vi "populate_database.vi"(11 "output cluster":T1) -> ()   [LabVIEW 2014]
uses:
  Program Files (x86)/National Instruments/LabVIEW 2014/vi.lib/addons/database/Connection.llb/DB Tools Open Connec (String).vi
  Program Files (x86)/National Instruments/LabVIEW 2014/vi.lib/addons/database/Connection.llb/Conn Execute.vi
  Program Files (x86)/National Instruments/LabVIEW 2014/vi.lib/addons/database/Recordset.llb/Rec Destroy - Connection.vi
  Program Files (x86)/National Instruments/LabVIEW 2014/vi.lib/addons/database/NI_Database_API.lvlib
panel:
  out "resulting string":string
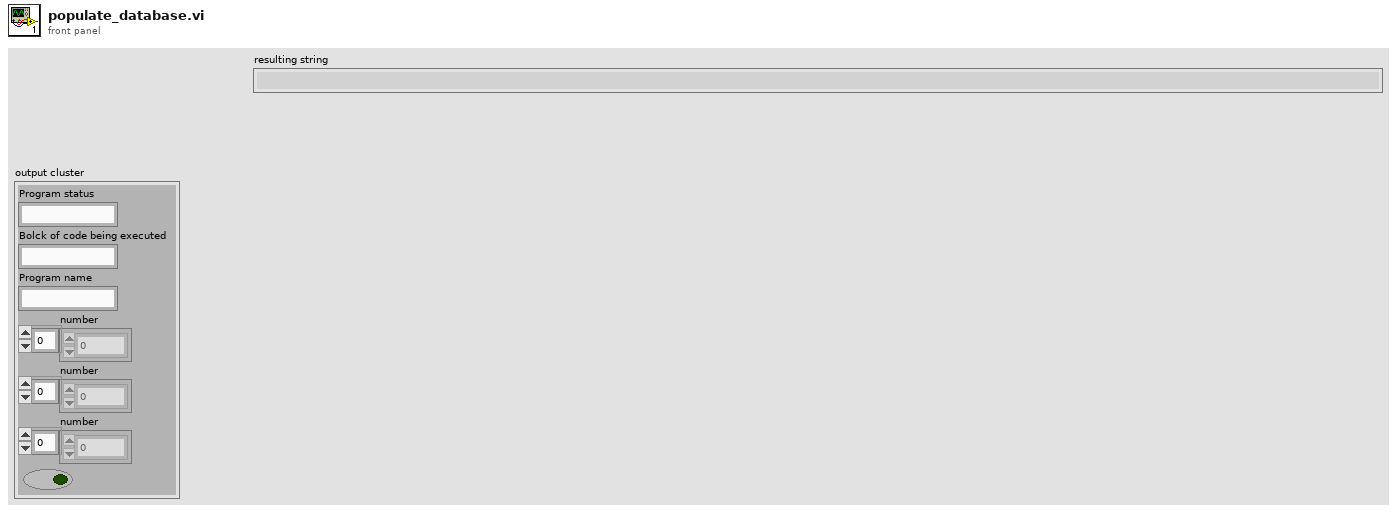
[diagram p1: front panel]
types:
  T1 = cluster{"Program status":string, "Bolck of code being executed":string, "Program name":string, "number":dbl[], "number":dbl[], "number":dbl[], bool}
  T2 = typedef "NI_Database_API.lvlib/Conn ObjectReference.ctl" = refnum<k1>
  T3 = typedef "NI_Database_API.lvlib/Rec ObjectReference.ctl" = refnum<k1>
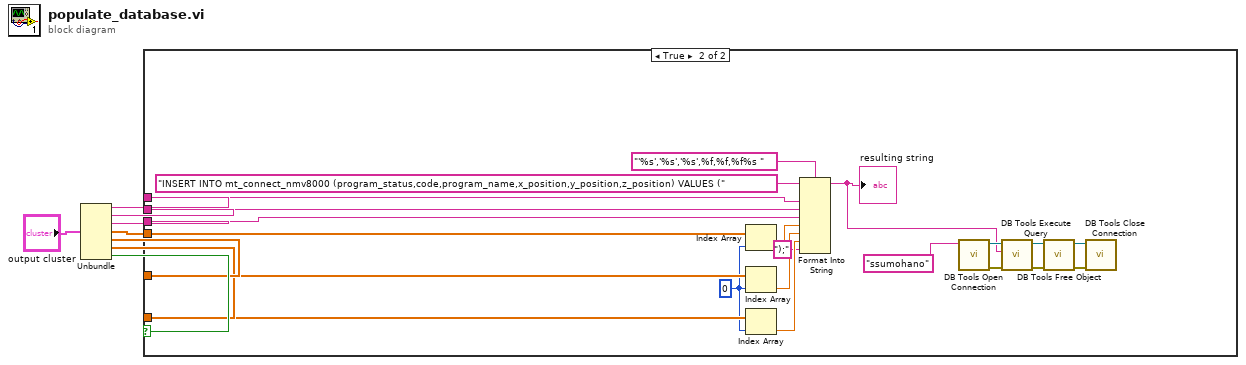
[diagram p0: block diagram]
diagram:
  n1 = Unbundle("output cluster") -> ("Program status"=w6:string, "Bolck of code being executed"=w5:string, "Program name"=w4:string, "number"=w3:dbl[], "number"=w2:dbl[], "number"=w1:dbl[], w7:bool)
  n2 = case shown="True" w7 {
    tunnel: w6 -> [_ w24]
    tunnel: w5 -> [_ w23]
    tunnel: w4 -> [_ w22]
    tunnel: w3 -> [_ w29]
    tunnel: w2 -> [_ w27]
    tunnel: w1 -> [_ w26]
    frame False {
    }
    frame True {
      w25 = 0 ("index")
      n3 = Index Array(array=w29, index=w25) -> (element=w21:dbl)
      n4 = Index Array(array=w27, index=w25) -> (element=w20:dbl)
      n5 = Index Array(array=w26, index=w25) -> (element=w19:dbl)
      n6 = Format Into String(format string="'%s','%s','%s',%f,%f,%f%s ", initial string="INSERT INTO mt_connect_nmv8000 (program_status,code,program_name,x_position,y_position,z_position) VALUES (", w24, w23, w22, w21, w20, w19, ");" ("input 7")) -> (resulting string=w9:string)  [unwired: 1 in, 1 out]
      "resulting string" <- w9
      n7 = call-poly "DB Tools Open Connection.vi"("connection information"="ssumohano") -> ("error out"=w14:errorcluster, "connection reference"=w15:T2)  [unwired: 7 in]
      n8 = call-poly "DB Tools Execute Query.vi"("error in (no error)"=w14, "SQL query"=w9, "connection reference"=w15) -> ("error out"=w13:errorcluster, "recordset reference"=w12:T3)  [unwired: 5 in]
      n9 = call-poly "DB Tools Free Object.vi"("error in (no error)"=w13, "recordset reference"=w12) -> ("error out"=w11:errorcluster, "connection reference"=w10:T2)  [unwired: 8 in]
      n10 = call "DB Tools Close Connection.vi"("error in (no error)"=w11, "connection reference"=w10) -> ()  [unwired: 5 in, 1 out]
    }
  }
